vi "SPIM control3d.vi"() -> ()   [LabVIEW 2012]
uses:
  Scanning Setting.vi
panel:
  in  "offset":dbl(slide) scale=0.0..-0.65
  out "Z-frequncy":dbl
  out "Z":dbl(slide)
  in  "Volum Scan":bool
  out "Trigger 4":dynamicdata(graph)=[{"t0"=timestamp(16448.7 s since 1904-01-01), "dt"=1e-05, "Y"=array[10000 elements], "attributes"=variant("NI_ChannelName"=variant(string "Triangle (Collected)"), "NI_ExpIsRelativeTime"=variant(bool TRUE), "NI_ExpStartTimeStamp"=variant(timestamp timestamp(3461934223.089551 s since 1904-01-01)), "NI_ExpTimeStamp"=variant(timestamp timestamp(3461934223.089551 s since 1904-01-01)), "NI_ExpXDimension"=variant(string "t"), "NI_OriginalChannelName"=variant(string "Triangle"))}, {"t0"=timestamp(16448.7 s since 1904-01-01), "dt"=1e-05, "Y"=array[10000 elements], "attributes"=variant("NI_ChannelName"=variant(string "Square (Collected)"), "NI_ExpIsRelativeTime"=variant(bool TRUE), "NI_ExpStartTimeStamp"=variant(timestamp timestamp(3461934223.089551 s since 1904-01-01)), "NI_ExpTimeStamp"=variant(timestamp timestamp(3461934223.089551 s since 1904-01-01)), "NI_ExpXDimension"=variant(string "t"), "NI_OriginalChannelName"=variant(string "Square"))}, {"t0"=timestamp(16448.7 s since 1904-01-01), "dt"=1e-05, "Y"=array[10000 elements], "attributes"=variant("NI_ChannelName"=variant(string "Square (Collected)"), "NI_ExpIsRelativeTime"=variant(bool TRUE), "NI_ExpStartTimeStamp"=variant(timestamp timestamp(3461934223.0885506 s since 1904-01-01)), "NI_ExpTimeStamp"=variant(timestamp timestamp(3461934223.0885506 s since 1904-01-01)), "NI_ExpXDimension"=variant(string "t"), "NI_OriginalChannelName"=variant(string "Square"))}]
  out "Trigger 3":dynamicdata(graph)=[{"t0"=timestamp(16448.7 s since 1904-01-01), "dt"=1e-05, "Y"=array[10000 elements], "attributes"=variant("NI_ChannelName"=variant(string "Triangle (Collected)"), "NI_ExpIsRelativeTime"=variant(bool TRUE), "NI_ExpStartTimeStamp"=variant(timestamp timestamp(3461934223.089551 s since 1904-01-01)), "NI_ExpTimeStamp"=variant(timestamp timestamp(3461934223.089551 s since 1904-01-01)), "NI_ExpXDimension"=variant(string "t"), "NI_OriginalChannelName"=variant(string "Triangle"))}, {"t0"=timestamp(16448.7 s since 1904-01-01), "dt"=1e-05, "Y"=array[10000 elements], "attributes"=variant("NI_ChannelName"=variant(string "Square (Collected)"), "NI_ExpIsRelativeTime"=variant(bool TRUE), "NI_ExpStartTimeStamp"=variant(timestamp timestamp(3461934223.089551 s since 1904-01-01)), "NI_ExpTimeStamp"=variant(timestamp timestamp(3461934223.089551 s since 1904-01-01)), "NI_ExpXDimension"=variant(string "t"), "NI_OriginalChannelName"=variant(string "Square"))}, {"t0"=timestamp(16448.7 s since 1904-01-01), "dt"=1e-05, "Y"=array[10000 elements], "attributes"=variant("NI_ChannelName"=variant(string "Square (Collected)"), "NI_ExpIsRelativeTime"=variant(bool TRUE), "NI_ExpStartTimeStamp"=variant(timestamp timestamp(3461934223.0885506 s since 1904-01-01)), "NI_ExpTimeStamp"=variant(timestamp timestamp(3461934223.0885506 s since 1904-01-01)), "NI_ExpXDimension"=variant(string "t"), "NI_OriginalChannelName"=variant(string "Square"))}]
  out "Trigger 2":dynamicdata(graph)=[{"t0"=timestamp(16448.7 s since 1904-01-01), "dt"=1e-05, "Y"=array[10000 elements], "attributes"=variant("NI_ChannelName"=variant(string "Triangle (Collected)"), "NI_ExpIsRelativeTime"=variant(bool TRUE), "NI_ExpStartTimeStamp"=variant(timestamp timestamp(3461934223.089551 s since 1904-01-01)), "NI_ExpTimeStamp"=variant(timestamp timestamp(3461934223.089551 s since 1904-01-01)), "NI_ExpXDimension"=variant(string "t"), "NI_OriginalChannelName"=variant(string "Triangle"))}, {"t0"=timestamp(16448.7 s since 1904-01-01), "dt"=1e-05, "Y"=array[10000 elements], "attributes"=variant("NI_ChannelName"=variant(string "Square (Collected)"), "NI_ExpIsRelativeTime"=variant(bool TRUE), "NI_ExpStartTimeStamp"=variant(timestamp timestamp(3461934223.089551 s since 1904-01-01)), "NI_ExpTimeStamp"=variant(timestamp timestamp(3461934223.089551 s since 1904-01-01)), "NI_ExpXDimension"=variant(string "t"), "NI_OriginalChannelName"=variant(string "Square"))}, {"t0"=timestamp(16448.7 s since 1904-01-01), "dt"=1e-05, "Y"=array[10000 elements], "attributes"=variant("NI_ChannelName"=variant(string "Square (Collected)"), "NI_ExpIsRelativeTime"=variant(bool TRUE), "NI_ExpStartTimeStamp"=variant(timestamp timestamp(3461934223.0885506 s since 1904-01-01)), "NI_ExpTimeStamp"=variant(timestamp timestamp(3461934223.0885506 s since 1904-01-01)), "NI_ExpXDimension"=variant(string "t"), "NI_OriginalChannelName"=variant(string "Square"))}]
  in  "1 Slice":bool
  in  "Structual":bool
  in  "Funcational":bool
  out "Peizo Voltage":dbl
  out "Peizo Location":dbl
  out "Z-Offset":dbl
  out "Scan Signal 2":cluster{"Y":dbl[], "Y":dbl[]}[](graph)
  out "Trigger":dynamicdata(graph)=[{"t0"=timestamp(16448.7 s since 1904-01-01), "dt"=1e-05, "Y"=array[10000 elements], "attributes"=variant("NI_ChannelName"=variant(string "Triangle (Collected)"), "NI_ExpIsRelativeTime"=variant(bool TRUE), "NI_ExpStartTimeStamp"=variant(timestamp timestamp(3461934223.089551 s since 1904-01-01)), "NI_ExpTimeStamp"=variant(timestamp timestamp(3461934223.089551 s since 1904-01-01)), "NI_ExpXDimension"=variant(string "t"), "NI_OriginalChannelName"=variant(string "Triangle"))}, {"t0"=timestamp(16448.7 s since 1904-01-01), "dt"=1e-05, "Y"=array[10000 elements], "attributes"=variant("NI_ChannelName"=variant(string "Square (Collected)"), "NI_ExpIsRelativeTime"=variant(bool TRUE), "NI_ExpStartTimeStamp"=variant(timestamp timestamp(3461934223.089551 s since 1904-01-01)), "NI_ExpTimeStamp"=variant(timestamp timestamp(3461934223.089551 s since 1904-01-01)), "NI_ExpXDimension"=variant(string "t"), "NI_OriginalChannelName"=variant(string "Square"))}, {"t0"=timestamp(16448.7 s since 1904-01-01), "dt"=1e-05, "Y"=array[10000 elements], "attributes"=variant("NI_ChannelName"=variant(string "Square (Collected)"), "NI_ExpIsRelativeTime"=variant(bool TRUE), "NI_ExpStartTimeStamp"=variant(timestamp timestamp(3461934223.0885506 s since 1904-01-01)), "NI_ExpTimeStamp"=variant(timestamp timestamp(3461934223.0885506 s since 1904-01-01)), "NI_ExpXDimension"=variant(string "t"), "NI_OriginalChannelName"=variant(string "Square"))}]
  out "Scan Signal":cluster{"Y":dbl[], "Y":dbl[]}[](graph)
  out "Error Out":errorcluster={"status"=TRUE, "code"=-200561, "source"="SPIM control.vi:Instance:14:1<append>\n<B>Data: </B>-10.007205\n<B>Specified Range Minimum: </B>-10.0\n<B>Specified Range Maximum: </B> 10.0\n\n<B>Task Name: </B>_unnamedTask<30>"}
  in  "Scanner":bool
  in  "Setting":bool
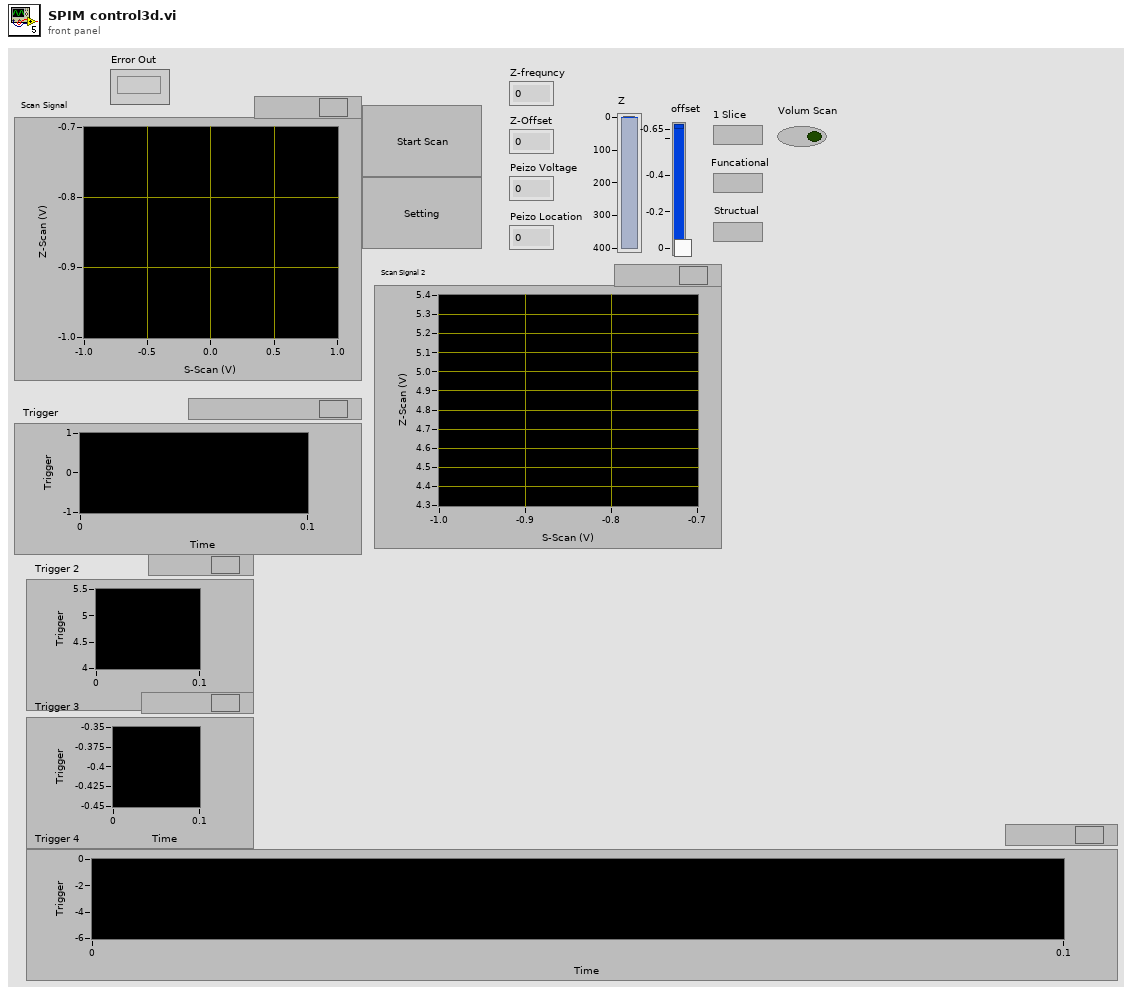
[diagram p1: front panel]
types:
  T1 = enum8{"Enabled", "Disabled", "Disabled and Grayed Out"}
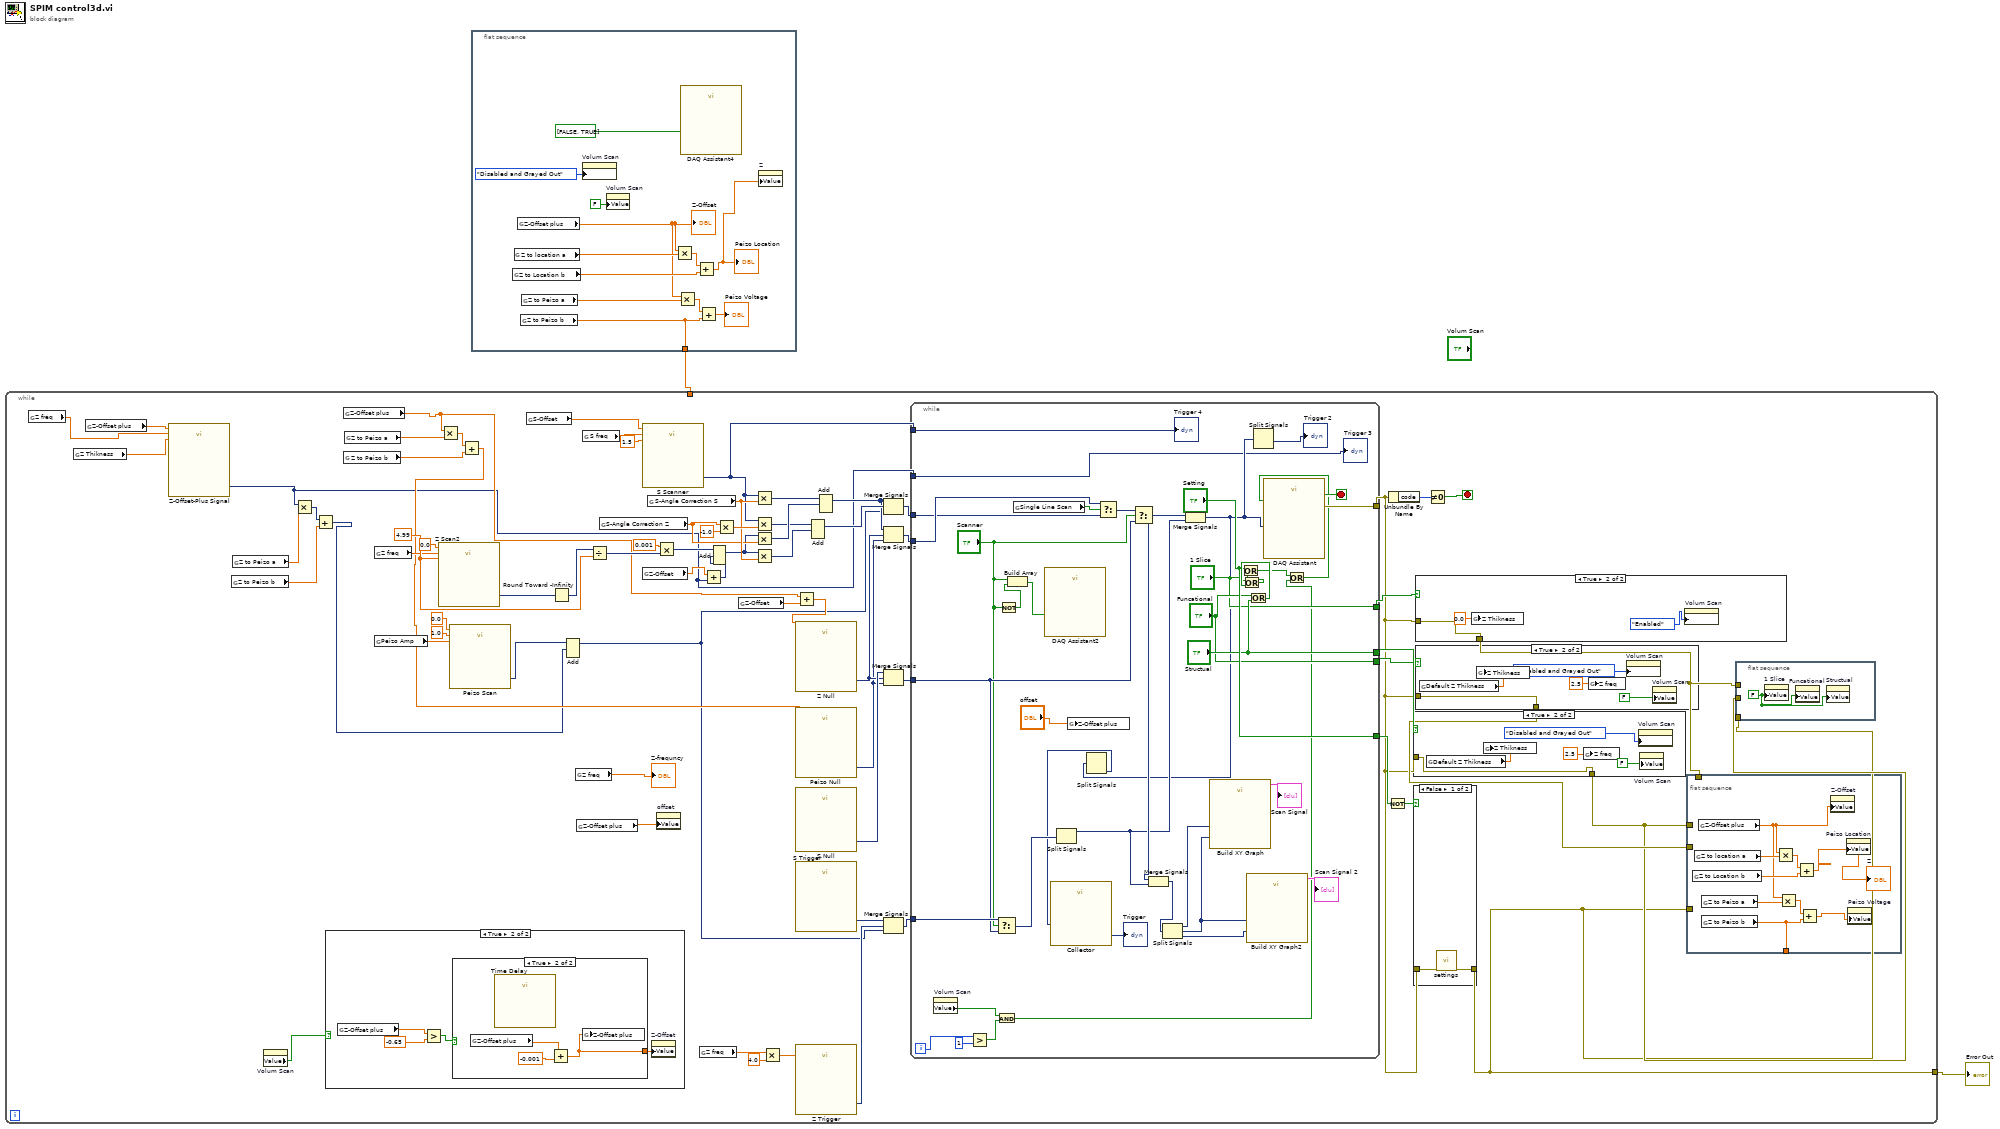
[diagram p0: block diagram]
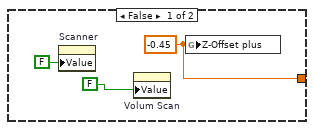
[diagram p3: hidden frame]
diagram:
  n1 = while {
    tunnel: [w9] -> w1
    tunnel: w2 -> [_]
    stop <- w48 stop-if-true
    w46 = 4.99 ("Amplitude")
    n2 = global read "Scanning Setting.vi" "Z freq"() -> (w18:dbl)
    n3 = global read "Scanning Setting.vi" "Z Thikness"() -> (w19:dbl)
    n4 = global read "Scanning Setting.vi" "Z-Offset plus"() -> (w27:dbl)
    n5 = call "Z-Offset-Plus Signal"("Offset"=w27, "Frequency"=w18, "Amplitude"=w19) -> ("Triangle"=w7:dynamicdata)  [unwired: 11 in, 1 out]
    n6 = global read "Scanning Setting.vi" "Z to Peizo b"() -> (w26:dbl)
    n7 = global read "Scanning Setting.vi" "Z to Peizo a"() -> (w25:dbl)
    n8 = property on="Volum Scan" class="Bool (strict)"() -> ("Value"=w5:bool)  [unwired: 2 in, 2 out]
    n9 = Multiply(x=w7, y=w25) -> (x*y=w24:dynamicdata)
    n10 = Add(x=w24, y=w26) -> (x+y=w22:dynamicdata)
    n11 = case shown="True" w5 {
      frame False {
      }
      frame True {
        n12 = global read "Scanning Setting.vi" "Z-Offset plus"() -> (w77:dbl)
        n13 = Greater?(x=w77, y=-0.65) -> (0:w78:bool)
        n14 = case shown="True" w78 {
          tunnel: [w80 w82] -> w75
          frame False {
            w80 = -0.45 ("Z-Offset plus")
            n15 = property on="Scanner" class="Bool (strict)"("Value"=FALSE ("Scanner")) -> ()  [unwired: 2 in, 2 out]
            n16 = property on="Volum Scan" class="Bool (strict)"("Value"=FALSE) -> ()  [unwired: 2 in, 2 out]
            n17 = global write "Scanning Setting.vi" "Z-Offset plus"(w80) -> ()
          }
          frame True {
            n18 = global read "Scanning Setting.vi" "Z-Offset plus"() -> (w83:dbl)
            n19 = call "Time Delay"() -> ()  [unwired: 11 in, 1 out]
            n20 = Add(x=w83, y=-0.001) -> (x+y=w82:dbl)
            n21 = global write "Scanning Setting.vi" "Z-Offset plus"(w82) -> ()
          }
        }
        n22 = property on="Z-Offset" class="DigNum (strict)"("Value"=w75) -> ()  [unwired: 2 in, 2 out]
      }
    }
    n23 = global read "Scanning Setting.vi" "Z-Offset plus"() -> (w28:dbl)
    n24 = global read "Scanning Setting.vi" "Z to Peizo b"() -> (w30:dbl)
    n25 = global read "Scanning Setting.vi" "Z to Peizo a"() -> (w31:dbl)
    n26 = global read "Scanning Setting.vi" "Peizo Amp"() -> (w38:dbl)
    n27 = global read "Scanning Setting.vi" "Z freq"() -> (w39:dbl)
    n28 = call "Z Scan2"("Offset"=0.0, "Frequency"=w39, "Amplitude"=w46) -> ("Triangle"=w43:dynamicdata)  [unwired: 11 in, 1 out]
    n29 = Multiply(x=w28, y=w31) -> (x*y=w32:dbl)
    n30 = call "Peizo Scan"("Offset"=0.0, "Frequency"=1.0, "Amplitude"=w38) -> ("Sine"=w23:dynamicdata)  [unwired: 11 in, 1 out]
    n31 = Add(x=w32, y=w30) -> (x+y=w29:dbl)
    n32 = global read "Scanning Setting.vi" "S-Offset"() -> (w62:dbl)
    n33 = Round Toward -Infinity(1:w43) -> (0:w44:dynamicdata)
    n34 = Add(1:w22, 2:w23) -> (0:w21:dynamicdata)  [unwired: 1 in, 1 out]
    n35 = global read "Scanning Setting.vi" "Z freq"() -> (→"Z-frequncy":dbl)
    n36 = global read "Scanning Setting.vi" "Z-Offset plus"() -> (w3:dbl)
    n37 = global read "Scanning Setting.vi" "S freq"() -> (w63:dbl)
    n38 = Divide(x=w44, y=w46) -> (x/y=w47:dynamicdata)
    n39 = global read "Scanning Setting.vi" "S-Angle Correction Z"() -> (w60:dbl)
    n40 = call "S Scanner"("Offset"=w62, "Frequency"=w63, "Amplitude"=1.5) -> ("Triangle"=w6:dynamicdata)  [unwired: 11 in, 1 out]
    n41 = global read "Scanning Setting.vi" "Z-Offset"() -> (w36:dbl)
    n42 = global read "Scanning Setting.vi" "S-Angle Correction S"() -> (w61:dbl)
    n43 = property on="offset" class="Slide (strict)"("Value"=w3) -> ()  [unwired: 2 in, 2 out]
    n44 = Multiply(x=0.001, y=w47) -> (x*y=w42:dynamicdata)
    n45 = global read "Scanning Setting.vi" "Z freq"() -> (w51:dbl)
    n46 = Add(x=w36, y=w7) -> (x+y=w35:dynamicdata)
    n47 = Add(1:w35, 2:w42) -> (0:w41:dynamicdata)  [unwired: 1 in, 1 out]
    n48 = Multiply(x=w60, y=-1.0) -> (x*y=w66:dbl)
    n49 = global read "Scanning Setting.vi" "Z-Offset"() -> (w34:dbl)
    n50 = Multiply(x=w6, y=w61) -> (x*y=w69:dynamicdata)
    n51 = Multiply(x=w6, y=w66) -> (x*y=w67:dynamicdata)
    n52 = Multiply(x=w41, y=w60) -> (x*y=w70:dynamicdata)
    n53 = Multiply(x=w41, y=w61) -> (x*y=w68:dynamicdata)
    n54 = Multiply(x=w51, y=4.0) -> (x*y=w52:dbl)
    n55 = call "Peizo Null"("Offset"=w29) -> ("Square"=w40:dynamicdata)  [unwired: 13 in, 1 out]
    n56 = call "S Null"() -> ("Triangle"=w74:dynamicdata)  [unwired: 14 in, 1 out]
    n57 = call "S Trigger"() -> ("Square"=w56:dynamicdata)  [unwired: 14 in, 1 out]
    n58 = call "Z Trigger"("Frequency"=w52) -> ("Square"=w55:dynamicdata)  [unwired: 13 in, 1 out]
    n59 = Add(x=w28, y=w34) -> (x+y=w33:dbl)
    n60 = call "Z Null"("Offset"=w33) -> ("Square"=w59:dynamicdata)  [unwired: 13 in, 1 out]
    n61 = Add(1:w68, 2:w67) -> (0:w64:dynamicdata)  [unwired: 1 in, 1 out]
    n62 = Add(1:w70, 2:w69) -> (0:w58:dynamicdata)  [unwired: 1 in, 1 out]
    n63 = Merge Signals(w58, w64, w21) -> (w73:dynamicdata)
    n64 = Merge Signals(w58, w59, w40) -> (w57:dynamicdata)
    n65 = Merge Signals(w74, w59, w40) -> (w72:dynamicdata)
    n66 = Merge Signals(w56, w55, w21) -> (w54:dynamicdata)
    n67 = while {
      tunnel: w73 -> [w148]
      tunnel: w72 -> [w143]
      tunnel: [w151] -> w8
      tunnel: w57 -> [w150]
      tunnel: w54 -> [w144]
      tunnel: ["Setting"] -> w16
      tunnel: ["Structual"] -> w15
      tunnel: ["Funcational"] -> w14
      tunnel: ["1 Slice"] -> w13
      tunnel: w7 -> [w123]
      tunnel: w6 -> [w122]
      i -> [w121]
      stop <- w153 stop-if-true
      n68 = property on="Volum Scan" class="Bool (strict)"() -> ("Value"=w118:bool)  [unwired: 2 in, 2 out]
      n69 = Greater?(x=w121, y=1) -> (0:w119:bool)
      n70 = Select(t=w144, s="Scanner", f=w143) -> (s? t:f=w138:dynamicdata)
      n71 = And(x=w118, y=w119) -> (x .and. y?=w115:bool)
      n72 = Not(x="Scanner") -> (.not. x?=w127:bool)
      n73 = Build Array("Scanner", w127) -> (w128:bool[])
      n74 = global read "Scanning Setting.vi" "Single Line Scan"() -> (w149:bool)
      n75 = call "DAQ Assistant2"("data"=w128) -> ()  [unwired: 17 in, 2 out]
      n76 = Split Signals(w138) -> (w135:dynamicdata)  [unwired: 3 in, 2 out]
      n77 = global write "Scanning Setting.vi" "Z-Offset plus"("offset") -> ()
      n78 = Select(t=w150, s=w149, f=w148) -> (s? t:f=w147:dynamicdata)
      n79 = Select(t=w147, s="Scanner", f=w143) -> (s? t:f=w146:dynamicdata)
      n80 = Merge Signals(w146, w135) -> (w136:dynamicdata)
      n81 = Split Signals(w136) -> (w140:dynamicdata, w141:dynamicdata, w139:dynamicdata)  [unwired: 3 in]
      n82 = Merge Signals(w146, w135) -> (w125:dynamicdata)
      n83 = Split Signals(w125) -> (w137:dynamicdata)  [unwired: 4 in, 3 out]
      n84 = call "Collector"("Signals"=w137) -> ("Collected Signals"=→"Trigger":dynamicdata)  [unwired: 9 in, 1 out]
      n85 = call "Build XY Graph"("Y Input"=w141, "X Input"=w140) -> ("XY Graph"=→"Scan Signal":cluster{"Y":dbl[], "Y":dbl[]}[])  [unwired: 3 in, 6 out]
      n86 = call "Build XY Graph2"("Y Input"=w139, "X Input"=w141) -> ("XY Graph"=→"Scan Signal 2":cluster{"Y":dbl[], "Y":dbl[]}[])  [unwired: 3 in, 6 out]
      n87 = Or(x="Funcational", y="Structual") -> (x .or. y?=w134:bool)
      n88 = Or(x="1 Slice", y=w134) -> (x .or. y?=w133:bool)
      n89 = Or(x="Setting", y=w133) -> (x .or. y?=w116:bool)
      n90 = Split Signals(w125) -> (→"Trigger 2":dynamicdata)  [unwired: 4 in, 3 out]
      n91 = Or(x=w116, y=w115) -> (x .or. y?=w117:bool)
      n92 = call "DAQ Assistant"("data"=w125, "stop (F)"=w117) -> ("stopped"=w153:bool, "error out"=w151:errorcluster)  [unwired: 15 in, 1 out]
      "Trigger 3" <- w123
      "Trigger 4" <- w122
    }
    n93 = Not(x=w16) -> (.not. x?=w17:bool)
    n94 = Unbundle By Name(w8) -> ("code"=w49:i32)
    n95 = case shown="True" w15 {
      tunnel: w8 -> [w96 w99]
      tunnel: [w96 w99] -> w10
      frame False {
      }
      frame True {
        n96 = global read "Scanning Setting.vi" "Default Z Thikness"() -> (w101:dbl)
        n97 = global write "Scanning Setting.vi" "Z Thikness"(w101) -> ()
        n98 = global write "Scanning Setting.vi" "Z freq"(2.5 ("Z freq")) -> ()
        n99 = property on="Volum Scan" class="Bool (strict)"("DisabledEnum"=T1."Disabled and Grayed Out" ("Disabled")) -> ()  [unwired: 2 in, 2 out]
        n100 = property on="Volum Scan" class="Bool (strict)"("Value"=FALSE ("Volum Scan")) -> ()  [unwired: 2 in, 2 out]
      }
    }
    n101 = case shown="False" w17 {
      tunnel: [w111 w113] -> w9
      tunnel: w8 -> [w112 w113]
      frame False {
        n102 = call "settings.vi"("Error In"=w112) -> ("Error Out"=w111:errorcluster)  [unwired: 10 in]
      }
      frame True {
      }
    }
    n103 = case shown="True" w13 {
      tunnel: w8 -> [w86 w88]
      tunnel: [w86 w88] -> w11
      frame False {
      }
      frame True {
        n104 = global write "Scanning Setting.vi" "Z Thikness"(0.0 ("Z Thikness")) -> ()
        n105 = property on="Volum Scan" class="Bool (strict)"("DisabledEnum"=T1."Enabled" ("Disabled")) -> ()  [unwired: 2 in, 2 out]
      }
    }
    n106 = case shown="True" w14 {
      tunnel: w8 -> [w90 w93]
      tunnel: [w90 w93] -> w12
      frame False {
      }
      frame True {
        n107 = global read "Scanning Setting.vi" "Default Z Thikness"() -> (w95:dbl)
        n108 = global write "Scanning Setting.vi" "Z Thikness"(w95) -> ()
        n109 = global write "Scanning Setting.vi" "Z freq"(2.5 ("Z freq")) -> ()
        n110 = property on="Volum Scan" class="Bool (strict)"("DisabledEnum"=T1."Disabled and Grayed Out" ("Disabled")) -> ()  [unwired: 2 in, 2 out]
        n111 = property on="Volum Scan" class="Bool (strict)"("Value"=FALSE ("Volum Scan")) -> ()  [unwired: 2 in, 2 out]
      }
    }
    n112 = Not Equal To 0?(x=w49) -> (x != 0?=w48:bool)
    n113 = flat-sequence {
      tunnel: [w105] -> _
      tunnel: w9 -> [_]
      tunnel: w10 -> [_]
      tunnel: w12 -> [_]
      tunnel: w11 -> [_]
      frame #0 {
        n114 = global read "Scanning Setting.vi" "Z to Location b"() -> (w108:dbl)
        n115 = global read "Scanning Setting.vi" "Z to location a"() -> (w110:dbl)
        n116 = global read "Scanning Setting.vi" "Z-Offset plus"() -> (w104:dbl)
        n117 = global read "Scanning Setting.vi" "Z to Peizo b"() -> (w105:dbl)
        n118 = global read "Scanning Setting.vi" "Z to Peizo a"() -> (w106:dbl)
        n119 = Multiply(x=w104, y=w110) -> (x*y=w109:dbl)
        n120 = Multiply(x=w104, y=w106) -> (x*y=w107:dbl)
        n121 = Add(x=w109, y=w108) -> (x+y=w102:dbl)
        "Z" <- w102
        n122 = Add(x=w107, y=w105) -> (x+y=w103:dbl)
        n123 = property on="Z-Offset" class="DigNum (strict)"("Value"=w104) -> ()  [unwired: 2 in, 2 out]
        n124 = property on="Peizo Location" class="DigNum (strict)"("Value"=w102) -> ()  [unwired: 2 in, 2 out]
        n125 = property on="Peizo Voltage" class="DigNum (strict)"("Value"=w103) -> ()  [unwired: 2 in, 2 out]
      }
    }
    n126 = flat-sequence {
      tunnel: w11 -> [_]
      tunnel: w10 -> [_]
      tunnel: w9 -> [_]
      frame #0 {
        w85 = FALSE ("1 Slice")
        n127 = property on="1 Slice" class="Bool (strict)"("Value"=w85) -> ()  [unwired: 2 in, 2 out]
        n128 = property on="Funcational" class="Bool (strict)"("Value"=w85) -> ()  [unwired: 2 in, 2 out]
        n129 = property on="Structual" class="Bool (strict)"("Value"=w85) -> ()  [unwired: 2 in, 2 out]
      }
    }
  }
  "Error Out" <- w1
  n130 = flat-sequence {
    tunnel: [w158] -> w2
    frame #0 {
      n131 = global read "Scanning Setting.vi" "Z to Location b"() -> (w163:dbl)
      n132 = global read "Scanning Setting.vi" "Z to location a"() -> (w165:dbl)
      n133 = global read "Scanning Setting.vi" "Z-Offset plus"() -> (w159:dbl)
      "Z-Offset" <- w159
      n134 = global read "Scanning Setting.vi" "Z to Peizo b"() -> (w158:dbl)
      n135 = global read "Scanning Setting.vi" "Z to Peizo a"() -> (w161:dbl)
      n136 = property on="Volum Scan" class="Bool (strict)"("DisabledEnum"=T1."Disabled and Grayed Out" ("Disabled")) -> ()  [unwired: 2 in, 2 out]
      n137 = property on="Volum Scan" class="Bool (strict)"("Value"=FALSE ("Volum Scan")) -> ()  [unwired: 2 in, 2 out]
      n138 = Multiply(x=w159, y=w165) -> (x*y=w164:dbl)
      n139 = Multiply(x=w159, y=w161) -> (x*y=w162:dbl)
      n140 = call "DAQ Assistant4"("data"=bool[] [FALSE, TRUE]) -> ()  [unwired: 17 in, 2 out]
      n141 = Add(x=w164, y=w163) -> (x+y=w154:dbl)
      "Peizo Location" <- w154
      n142 = Add(x=w162, y=w158) -> (x+y=→"Peizo Voltage":dbl)
      n143 = property on="Z" class="Slide (strict)"("Value"=w154) -> ()  [unwired: 2 in, 2 out]
    }
  }
